vi "1D Convolution (DBL).vi"(9 "algorithm":enum32{"direct", "frequency domain"}(ring)=enum."frequency domain", 10 "Y":dbl[](array[numeric]), 11 "X":dbl[](array[numeric])) -> (0 "error":i32, 3 "X * Y":dbl[](array[numeric]))   [LabVIEW 2017, in "NI_AALPro.lvlib"]
doc: "Computes the convolution of the input sequences <B>X</B> and <B>Y</B>. Wire data to the <B>X</B> and <B>Y</B> inputs to determine the polymorphic instance to use or manually select the instance."
uses:
  NI_AALPro.lvlib
  lvanlys.dll
panel:
  # "1D Convolution (DBL)"
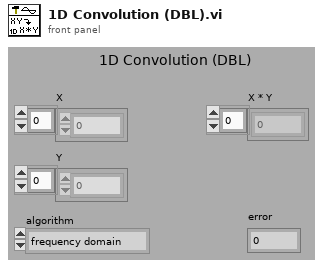
[diagram p1: front panel]
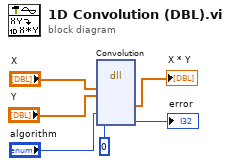
[diagram p0: block diagram]
diagram:
  n1 = dll-call lib="C:/Program Files/National Instruments/LabVIEW 2017/resource/lvanlys.*" fn="Convolution"("X"="X", "Y"="Y", "algorithm"="algorithm", "error"=0) -> ("X * Y"=→"X * Y":dbl[], "error"=→"error":i32)  [unwired: 8 in, 2 out]
